vi "Create Template Sources.vi"() -> ()   [LabVIEW 2014]
uses:
  <vilib>/vision/NI_Vision_Development_Module.lvlib
panel:
  out "Image":T1(plugin-control)
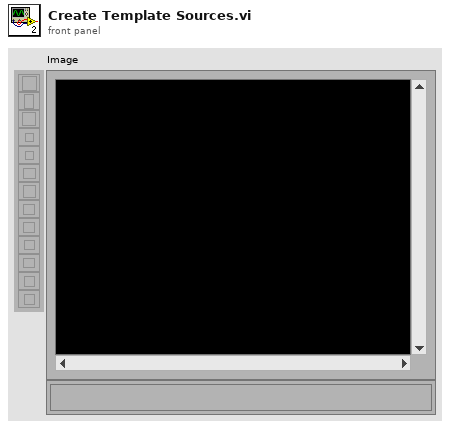
[diagram p1: front panel]
types:
  T1 = typedef "IMAQ Image.ctl" = refnum<image>
  T2 = typedef "Image Type" = u32
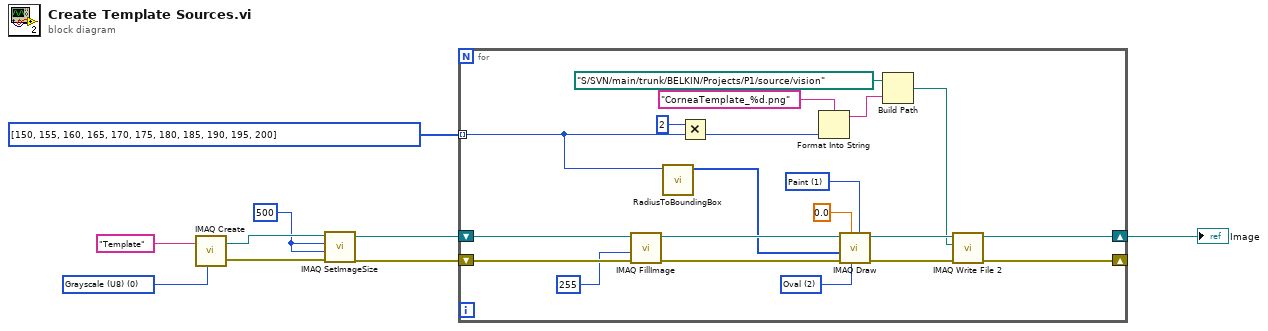
[diagram p0: block diagram]
diagram:
  w6 = 500 ("X Resolution")
  w9 = T2 0 items=["Grayscale (U8)", "Grayscale (I16)", "Grayscale (SGL)", "Complex (CSG)", "RGB (U32)", "HSL (U32)", "RGB (U64)", "Grayscale (U16)"] ("Image Type")
  n1 = call "IMAQ Create"("Image Name"="Template", "Image Type"=w9) -> ("New Image"=w7:T1, "error out"=w5:errorcluster)  [unwired: 3 in]
  n2 = call "IMAQ SetImageSize"("error in (no error)"=w5, "Y Resolution"=w6, "X Resolution"=w6, "Image"=w7) -> ("error out"=w3:errorcluster, "Image Out"=w4:T1)  [unwired: 1 in]
  n3 = for {
    shift-right: [w18] -> w2
    shift-left: w4 -> [w29]
    tunnel: i32[] [150, 155, 160, 165, 170, 175, 180, 185, 190, 195, 200] -> [w15] mode=indexing
    shift-right: [w12] -> _
    shift-left: w3 -> [w28]
    w21 = u16 1 items=["Frame", "Paint", "Invert Frame", "Invert Paint"] ("Draw Mode")
    w24 = u16 2 items=["Line", "Rectangle", "Oval"] ("Shape to draw")
    n4 = call "IMAQ FillImage"("error in (no error)"=w28, "Pixel Value (U8, U16, I16, Float)"=u8 255, "Image"=w29) -> ("error out"=w25:errorcluster, "Image Out"=w26:T1)  [unwired: 7 in]
    n5 = call "RadiusToBoundingBox.vi"("Radius"=w15) -> ("Array"=w22:i32[])  [unwired: 10 in]
    n6 = Multiply(x=2, y=w15) -> (x*y=w11:i32)
    n7 = Format Into String(format string="CorneaTemplate_%d.png" ("name or relative path"), w11) -> (resulting string=w16:string)  [unwired: 2 in, 1 out]
    n8 = call "IMAQ Draw"("Draw Mode"=w21, "Shape to draw"=w24, "Pixel Color"=sgl 0.0, "error in (no error)"=w25, "Coordinates"=w22, "Image Src"=w26) -> ("error out"=w19:errorcluster, "Image Dst Out"=w20:T1)  [unwired: 4 in]
    n9 = Build Path(base path=path "S:/SVN/main/trunk/BELKIN/Projects/P1/source/vision", name or relative path=w16) -> (appended path=w14:path)
    n10 = call-poly "IMAQ Write File 2"("error in (no error)"=w19, "File Path"=w14, "Image"=w20) -> ("error out"=w12:errorcluster, "Image Out (duplicate)"=w18:T1)  [unwired: 7 in]
  }
  "Image" <- w2
